vi "Do Query.vi"(9 "Query Builder":refnum<class "Query Builder.lvclass">, 11 "Database in":refnum<class "Database Platform.lvclass">) -> (0 "error out":errorcluster, 2 "Results":refnum<class "Result Row.lvclass">[](array[class]), 3 "Database out":refnum<class "Database Platform.lvclass">)   [LabVIEW 2020, in "Conditu2.lvlib" / "Database Platform.lvclass"]
uses:
  Database Platform.lvclass
  Query Builder/Query Builder.lvclass
  Result Row/Result Row.lvclass
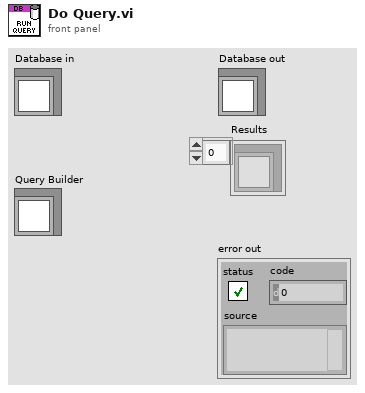
[diagram p1: front panel]
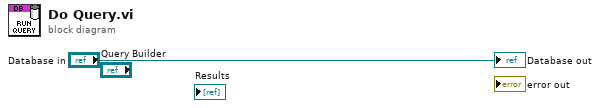
[diagram p0: block diagram]
diagram:
  "Database out" <- "Database in"
